vi "ExternalOUT.vi"(0 "nDeviceNo":u32, 1 "Mode":u16(ring) items=["Get&Set", "Get", "Set"], 5 "nChildNo":u32, 9 "NewExternalOutMode":u32[](array[numeric]), 11 "Error_In":T1) -> (2 "ExternalOut1ModeList":cluster{string, i32}[](array[cluster]), 3 "ExternalOut2ModeList":cluster{string, i32}[](array[cluster]), 4 "Error?":bool, 6 "ExternalOut1Mode":u32, 8 "ExternalOut2Mode":u32, 10 "ExternalOut3Mode":u32, 12 "ExternalOut3ModeList":cluster{string, i32}[](array[cluster]), 13 "ExternalOut4ModeList":cluster{string, i32}[](array[cluster]), 14 "ExternalOut4Mode":u32, 15 "Error_Out":T1)   [LabVIEW 2015]
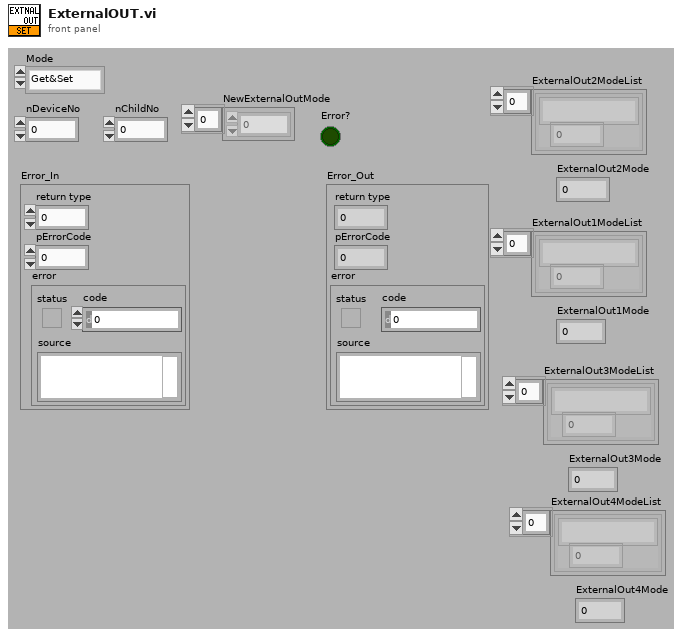
[diagram p1: front panel]
types:
  T1 = cluster{"return type":u32, "pErrorCode":u32, "error ":errorcluster}
  T2 = cluster{"ReturnValue":u32, "ErrorCode":u32, "error ":errorcluster}
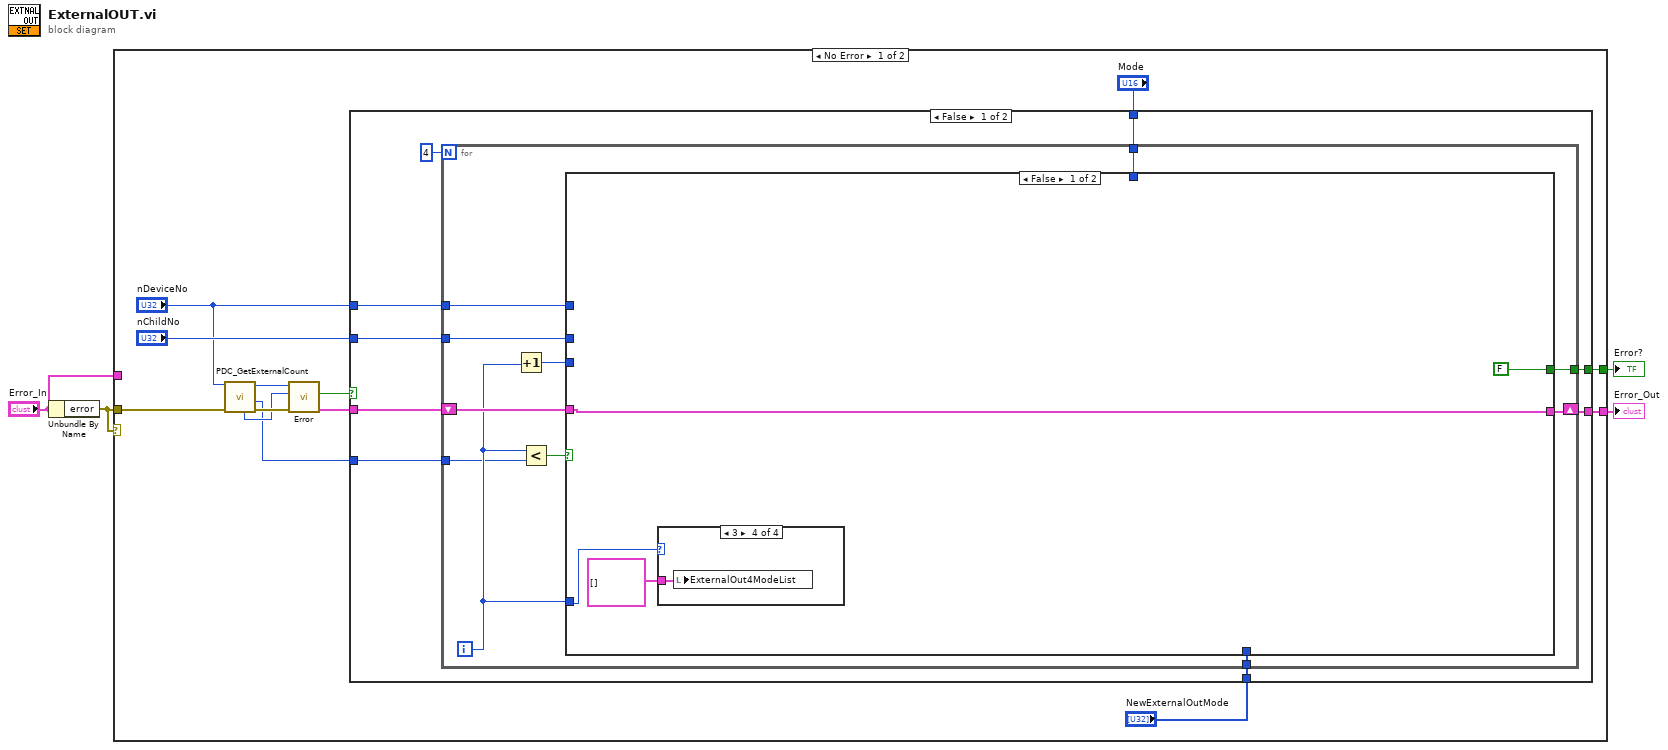
[diagram p0: block diagram]
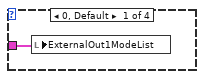
[diagram p2: hidden frame]
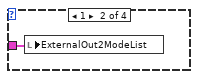
[diagram p3: hidden frame]
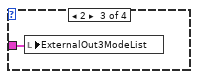
[diagram p4: hidden frame]
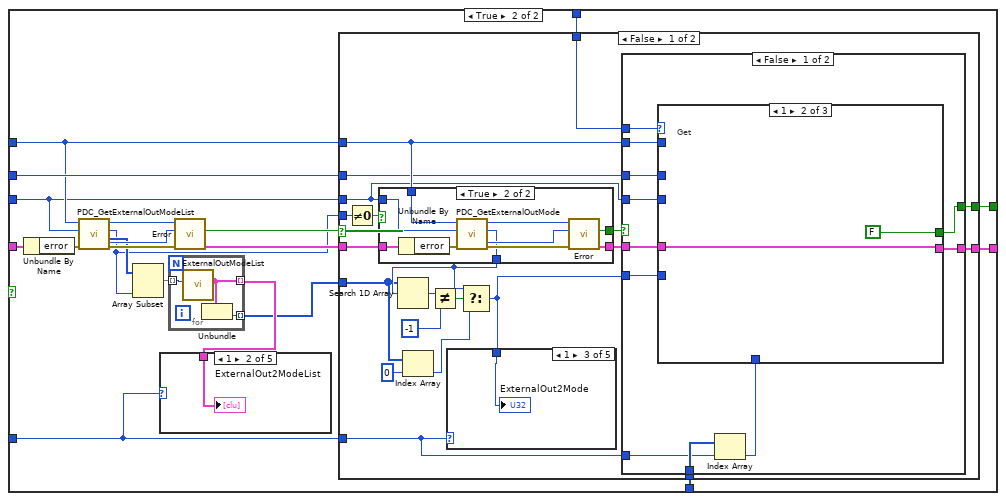
[diagram p5: hidden frame]
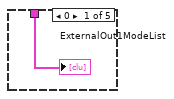
[diagram p6: hidden frame]
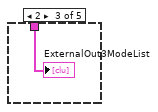
[diagram p7: hidden frame]
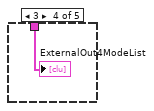
[diagram p8: hidden frame]
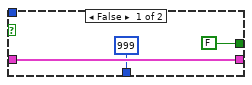
[diagram p10: hidden frame]
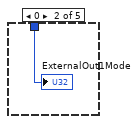
[diagram p12: hidden frame]
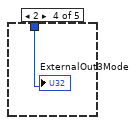
[diagram p13: hidden frame]
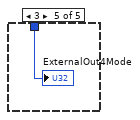
[diagram p14: hidden frame]
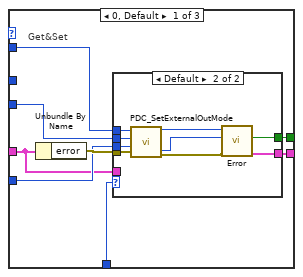
[diagram p15: hidden frame]
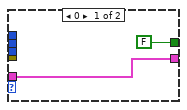
[diagram p16: hidden frame]
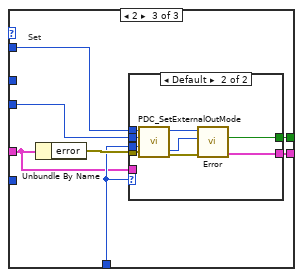
[diagram p17: hidden frame]
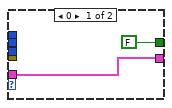
[diagram p18: hidden frame]
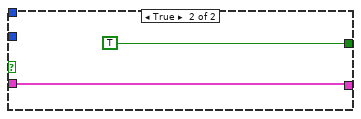
[diagram p19: hidden frame]
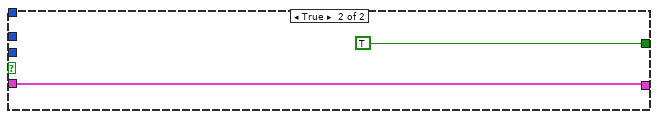
[diagram p20: hidden frame]
diagram:
  n1 = Unbundle By Name("Error_In") -> ("error"=w2:errorcluster)
  n2 = case shown="No Error" w2 {
    tunnel: [w17 w168] -> w4
    tunnel: [w16 TRUE ("Error?")] -> w3
    tunnel: w2 -> [w9 _]
    tunnel: "Error_In" -> [_ w168]
    frame No Error {
      n3 = call "PDC_GetExternalCount.vi"("error in (no error)"=w9, "DeviceNo"="nDeviceNo") -> ("error out"=w10:errorcluster, "Out"=w5:u32, "ReturnValue"=w8:u32, "ErrorCode"=w6:u32)  [unwired: 6 out]
      n4 = call "Error.vi"("error in (no error)"=w10, "ErrorCode"=w6, "ReturnValue"=w8) -> ("Error_Out"=w12:T2, "Error?"=w13:bool)  [unwired: 7 out]
      n5 = case shown="False" w13 {
        tunnel: [w26 w165] -> w17
        tunnel: [w25 TRUE ("Error?")] -> w16
        tunnel: "nChildNo" -> [w24 _]
        tunnel: "nDeviceNo" -> [w21 _]
        tunnel: "Mode" -> [w23 _]
        tunnel: w12 -> [w19 w165]
        tunnel: "NewExternalOutMode" -> [w22 _]
        tunnel: w5 -> [w18 _]
        frame False {
          n6 = for {
            N: 4 -> [_]
            tunnel: [w36] -> w25
            tunnel: w24 -> [w35]
            tunnel: w21 -> [w34]
            tunnel: w23 -> [w33]
            shift-right: [w37] -> w26
            shift-left: w19 -> [w32]
            tunnel: w22 -> [w31]
            tunnel: w18 -> [w27]
            i -> [w28]
            n7 = Increment(x=w28) -> (x+1=w30:i32)
            n8 = Less?(x=w28, y=w27) -> (x < y?=w29:bool)
            n9 = case shown="False" w29 {
              tunnel: [w41 w65] -> w37
              tunnel: [FALSE ("Error?") w64] -> w36
              tunnel: w35 -> [_ w63]
              tunnel: w34 -> [_ w55]
              tunnel: w33 -> [_ w53]
              tunnel: w32 -> [w41 w52]
              tunnel: w28 -> [w39 w50]
              tunnel: w30 -> [_ w49]
              tunnel: w31 -> [_ w48]
              frame False {
                n10 = case shown="3" w39 {
                  tunnel: cluster{string, i32}[] [] ("External\nGeneralOutModeList") -> [w42 w43 w44 w45]
                  frame 0, Default {
                    n11 = local write "ExternalOut1ModeList"(w42) -> ()
                  }
                  frame 1 {
                    n12 = local write "ExternalOut2ModeList"(w43) -> ()
                  }
                  frame 2 {
                    n13 = local write "ExternalOut3ModeList"(w44) -> ()
                  }
                  frame 3 {
                    n14 = local write "ExternalOut4ModeList"(w45) -> ()
                  }
                }
              }
              frame True {
                n15 = Unbundle By Name(w52) -> ("error"=w51:errorcluster)
                n16 = call "PDC_GetExternalOutModeList.vi"("error in (no error)"=w51, "PortNo"=w49, "DeviceNo"=w55) -> ("error out"=w62:errorcluster, "List"=w58:u32[], "Size"=w46:u32, "ReturnValue"=w61:u32, "ErrorCode"=w60:u32)  [unwired: 4 out]
                n17 = Array Subset(array=w58, length=w46) -> (w59:u32[])  [unwired: 1 in]
                n18 = for {
                  tunnel: w59 -> [w164] mode=indexing
                  tunnel: [w163] -> w57 mode=indexing
                  tunnel: [w162] -> w47 mode=indexing
                  n19 = call "ExternalOutModeList.vi"("List"=w164) -> ("GetLUTModeList"=w163:cluster{string, i32})  [unwired: 10 out]
                  n20 = Unbundle(w163) -> (w162:i32)  [unwired: 1 out]
                }
                n21 = case shown="1" w50 {
                  tunnel: w57 -> [w66 w67 w68 w69 _]
                  frame 0 {
                    "ExternalOut1ModeList" <- w66
                  }
                  frame 1 {
                    "ExternalOut2ModeList" <- w67
                  }
                  frame 2 {
                    "ExternalOut3ModeList" <- w68
                  }
                  frame 3 {
                    "ExternalOut4ModeList" <- w69
                  }
                  frame Default {
                  }
                }
                n22 = call "Error.vi"("error in (no error)"=w62, "ErrorCode"=w60, "ReturnValue"=w61) -> ("Error_Out"=w56:T2, "Error?"=w54:bool)  [unwired: 7 out]
                n23 = case shown="False" w54 {
                  tunnel: [w88 w161] -> w65
                  tunnel: [w87 TRUE ("Error?")] -> w64
                  tunnel: w56 -> [w86 w161]
                  tunnel: w55 -> [w85 _]
                  tunnel: w63 -> [w84 _]
                  tunnel: w49 -> [w72 _]
                  tunnel: w53 -> [w83 _]
                  tunnel: w50 -> [w81 _]
                  tunnel: w48 -> [w82 _]
                  tunnel: w47 -> [w75 _]
                  tunnel: w46 -> [w71 _]
                  frame False {
                    n24 = Not Equal To 0?(x=w71) -> (x != 0?=w70:bool)
                    n25 = case shown="True" w70 {
                      tunnel: [FALSE ("Error?") w100] -> w90
                      tunnel: [w92 w99] -> w89
                      tunnel: w86 -> [w92 w97]
                      tunnel: w85 -> [_ w96]
                      tunnel: w72 -> [_ w95]
                      tunnel: [u32 999 ("pMode") w94] -> w77
                      frame False {
                      }
                      frame True {
                        n26 = Unbundle By Name(w97) -> ("error"=w98:errorcluster)
                        n27 = call "PDC_GetExternalOutMode.vi"("error in (no error)"=w98, "Port"=w95, "DeviceNo"=w96) -> ("error out"=w101:errorcluster, "Mode"=w94:u32, "ReturnValue"=w102:u32, "ErrorCode"=w103:u32)  [unwired: 5 out]
                        n28 = call "Error.vi"("error in (no error)"=w101, "ErrorCode"=w103, "ReturnValue"=w102) -> ("Error_Out"=w99:T2, "Error?"=w100:bool)  [unwired: 7 out]
                      }
                    }
                    n29 = Search 1D Array(1D array=w75, element=w77) -> (index of element=w80:i32)  [unwired: 1 out]
                    n30 = Index Array(array=w75, index=0 ("指標")) -> (element=w73:i32)
                    n31 = Not Equal?(x=w80, y=-1) -> (x != y?=w78:bool)
                    n32 = Select(t=w77, s=w78, f=w73) -> (s? t:f=w76:u32)
                    n33 = case shown="1" w81 {
                      tunnel: w76 -> [_ w104 w105 w106 w107]
                      frame Default {
                      }
                      frame 0 {
                        "ExternalOut1Mode" <- w104
                      }
                      frame 1 {
                        "ExternalOut2Mode" <- w105
                      }
                      frame 2 {
                        "ExternalOut3Mode" <- w106
                      }
                      frame 3 {
                        "ExternalOut4Mode" <- w107
                      }
                    }
                    n34 = case shown="False" w90 {
                      tunnel: w89 -> [w112 w159]
                      tunnel: [w118 w159] -> w88
                      tunnel: w85 -> [w115 _]
                      tunnel: w84 -> [w114 _]
                      tunnel: [w117 TRUE ("Error?")] -> w87
                      tunnel: w83 -> [w116 _]
                      tunnel: w76 -> [w113 _]
                      tunnel: w72 -> [w111 _]
                      tunnel: w82 -> [w110 _]
                      tunnel: w81 -> [w109 _]
                      frame False {
                        n35 = Index Array(array=w110, index=w109) -> (element=w108:u32)
                        n36 = case shown="1" w116 {
                          tunnel: w112 -> [w119 w139 w140]
                          tunnel: [w125 w139 w145] -> w118
                          tunnel: w115 -> [w124 _ w144]
                          tunnel: w114 -> [_ _ _]
                          tunnel: [w123 FALSE ("Error?") w143] -> w117
                          tunnel: w113 -> [w122 _ _]
                          tunnel: w111 -> [w121 _ w142]
                          tunnel: w108 -> [w120 _ w141]
                          frame 0, Default {
                            # "Get&Set"
                            n37 = Unbundle By Name(w119) -> ("error"=w126:errorcluster)
                            n38 = case shown="Default" w120 {
                              tunnel: w126 -> [_ w137]
                              tunnel: [w128 w133] -> w125
                              tunnel: w124 -> [_ w132]
                              tunnel: [FALSE ("Error?") w131] -> w123
                              tunnel: w122 -> [_ w130]
                              tunnel: w121 -> [_ w129]
                              tunnel: w119 -> [w128 _]
                              frame 0 {
                              }
                              frame Default {
                                n39 = call "PDC_SetExternalOutMode.vi"("error in (no error)"=w137, "Mode"=w130, "Port"=w129, "DeviceNo"=w132) -> ("error out"=w134:errorcluster, "ReturnValue"=w136:u32, "ErrorCode"=w135:u32)  [unwired: 5 out]
                                n40 = call "Error.vi"("error in (no error)"=w134, "ErrorCode"=w135, "ReturnValue"=w136) -> ("Error_Out"=w133:T2, "Error?"=w131:bool)  [unwired: 7 out]
                              }
                            }
                          }
                          frame 1 {
                            # "Get"
                          }
                          frame 2 {
                            # "Set"
                            n41 = Unbundle By Name(w140) -> ("error"=w146:errorcluster)
                            n42 = case shown="Default" w141 {
                              tunnel: w146 -> [_ w157]
                              tunnel: [w148 w153] -> w145
                              tunnel: w144 -> [_ w152]
                              tunnel: [FALSE ("Error?") w151] -> w143
                              tunnel: w142 -> [_ w150]
                              tunnel: w141 -> [_ w149]
                              tunnel: w140 -> [w148 _]
                              frame 0 {
                              }
                              frame Default {
                                n43 = call "PDC_SetExternalOutMode.vi"("error in (no error)"=w157, "Mode"=w149, "Port"=w150, "DeviceNo"=w152) -> ("error out"=w154:errorcluster, "ReturnValue"=w156:u32, "ErrorCode"=w155:u32)  [unwired: 5 out]
                                n44 = call "Error.vi"("error in (no error)"=w154, "ErrorCode"=w155, "ReturnValue"=w156) -> ("Error_Out"=w153:T2, "Error?"=w151:bool)  [unwired: 7 out]
                              }
                            }
                          }
                        }
                      }
                      frame True {
                      }
                    }
                  }
                  frame True {
                  }
                }
              }
            }
          }
        }
        frame True {
        }
      }
    }
    frame Error {
    }
  }
  "Error_Out" <- w4
  "Error?" <- w3
